vi "set_ai_power.vi"(11 "pow":i32) -> ()   [LabVIEW 2012]
uses:
  <vilib>/Embedded/WSN/EIO/NI WSN-3202/EIO Prop Node Sensor Excitation Mode.ctl
  <vilib>/eio/EIOPropertyNode/EIOPropertyNode.xnode
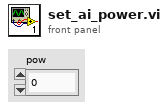
[diagram p1: front panel]
types:
  T1 = typedef "EIO Prop Node Sensor Excitation Mode.ctl" = u16
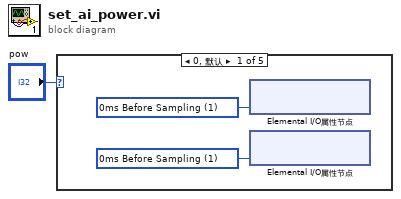
[diagram p0: block diagram]
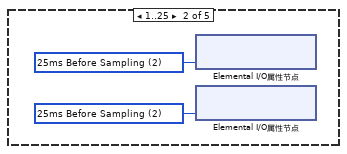
[diagram p2: hidden frame]
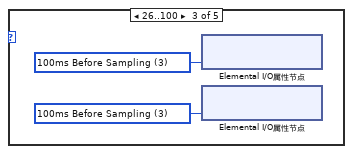
[diagram p3: hidden frame]
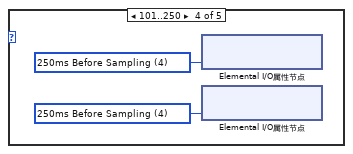
[diagram p4: hidden frame]
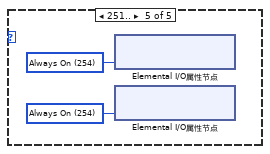
[diagram p5: hidden frame]
diagram:
  n1 = case shown="0, 默认" "pow" {
    frame 0, Default {
      w2 = T1 1 items=["Host Driven"=65535, "0ms Before Sampling"=1, "25ms Before Sampling"=2, "100ms Before Sampling"=3, "250ms Before Sampling"=4, "Always On"=254] ("Sensor Power")
      w3 = T1 1 items=["Host Driven"=65535, "0ms Before Sampling"=1, "25ms Before Sampling"=2, "100ms Before Sampling"=3, "250ms Before Sampling"=4, "Always On"=254] ("Sensor Power")
      n2 = xnode "Elemental I/O属性节点"("Sensor Power"=w2) -> ()  [unwired: 1 in, 1 out]
      n3 = xnode "Elemental I/O属性节点"("Sensor Power"=w3) -> ()  [unwired: 1 in, 1 out]
    }
    frame 1..25 {
      w8 = T1 2 items=["Host Driven"=65535, "0ms Before Sampling"=1, "25ms Before Sampling"=2, "100ms Before Sampling"=3, "250ms Before Sampling"=4, "Always On"=254] ("Sensor Power")
      w9 = T1 2 items=["Host Driven"=65535, "0ms Before Sampling"=1, "25ms Before Sampling"=2, "100ms Before Sampling"=3, "250ms Before Sampling"=4, "Always On"=254] ("Sensor Power")
      n4 = xnode "Elemental I/O属性节点"("Sensor Power"=w8) -> ()  [unwired: 1 in, 1 out]
      n5 = xnode "Elemental I/O属性节点"("Sensor Power"=w9) -> ()  [unwired: 1 in, 1 out]
    }
    frame 26..100 {
      w14 = T1 3 items=["Host Driven"=65535, "0ms Before Sampling"=1, "25ms Before Sampling"=2, "100ms Before Sampling"=3, "250ms Before Sampling"=4, "Always On"=254] ("Sensor Power")
      w15 = T1 3 items=["Host Driven"=65535, "0ms Before Sampling"=1, "25ms Before Sampling"=2, "100ms Before Sampling"=3, "250ms Before Sampling"=4, "Always On"=254] ("Sensor Power")
      n6 = xnode "Elemental I/O属性节点"("Sensor Power"=w14) -> ()  [unwired: 1 in, 1 out]
      n7 = xnode "Elemental I/O属性节点"("Sensor Power"=w15) -> ()  [unwired: 1 in, 1 out]
    }
    frame 101..250 {
      w20 = T1 4 items=["Host Driven"=65535, "0ms Before Sampling"=1, "25ms Before Sampling"=2, "100ms Before Sampling"=3, "250ms Before Sampling"=4, "Always On"=254] ("Sensor Power")
      w21 = T1 4 items=["Host Driven"=65535, "0ms Before Sampling"=1, "25ms Before Sampling"=2, "100ms Before Sampling"=3, "250ms Before Sampling"=4, "Always On"=254] ("Sensor Power")
      n8 = xnode "Elemental I/O属性节点"("Sensor Power"=w20) -> ()  [unwired: 1 in, 1 out]
      n9 = xnode "Elemental I/O属性节点"("Sensor Power"=w21) -> ()  [unwired: 1 in, 1 out]
    }
    frame 251.. {
      w26 = T1 254 items=["Host Driven"=65535, "0ms Before Sampling"=1, "25ms Before Sampling"=2, "100ms Before Sampling"=3, "250ms Before Sampling"=4, "Always On"=254] ("Sensor Power")
      w27 = T1 254 items=["Host Driven"=65535, "0ms Before Sampling"=1, "25ms Before Sampling"=2, "100ms Before Sampling"=3, "250ms Before Sampling"=4, "Always On"=254] ("Sensor Power")
      n10 = xnode "Elemental I/O属性节点"("Sensor Power"=w26) -> ()  [unwired: 1 in, 1 out]
      n11 = xnode "Elemental I/O属性节点"("Sensor Power"=w27) -> ()  [unwired: 1 in, 1 out]
    }
  }
